vi "Create Weather Display Objects.vi"(8 "Error In":errorcluster, 11 "Display Manager In":refnum<class "Display Manager.lvclass">) -> (0 "Error Out":errorcluster, 3 "Display Manager Out":refnum<class "Display Manager.lvclass">)   [LabVIEW 2021, in "Display Manager.lvclass"]
uses:
  Display Manager.lvclass
  <vilib>/Memosfet/myRIO-Neopixel/RT/Display Utilities/Public/Controls/2D Coordinates.ctl
  <vilib>/Memosfet/myRIO-Neopixel/RT/String/String.lvclass
  C:/Program Files (x86)/National Instruments/LabVIEW 2021/vi.lib/Memosfet/myRIO-Neopixel/RT/Display Element/Display Element.lvclass
  Accessors/Display/Get Display.vi
  <vilib>/Memosfet/myRIO-Neopixel/RT/Display/Display.lvclass
  <vilib>/Memosfet/myRIO-Neopixel/RT/Display Utilities/Display Utilities.lvlib
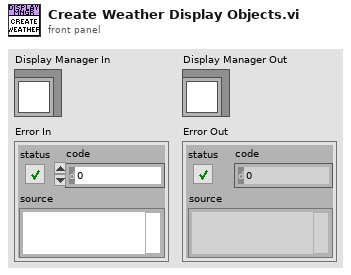
[diagram p1: front panel]
types:
  T1 = typedef "Display Utilities.lvlib/2D Coordinates.ctl" = cluster{"X":i32, "Y":i32}
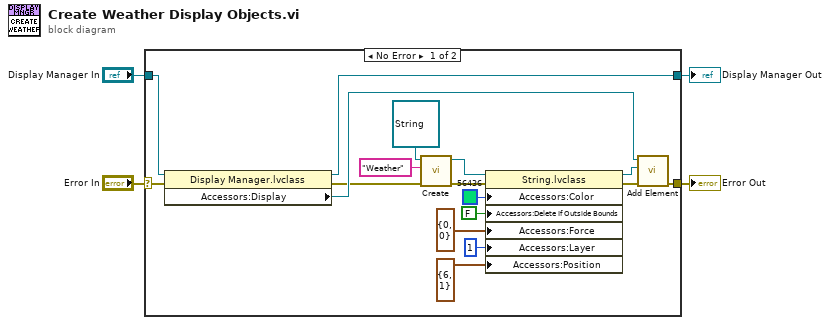
[diagram p0: block diagram]
diagram:
  n1 = case shown="No Error" "Error In" {
    selector: "Error In" -> [w20 w23]
    tunnel: [w6 w23] -> w3
    tunnel: "Display Manager In" -> [w21 w22]
    tunnel: [w17 w22] -> w1
    frame No Error {
      n2 = property class="Display Manager.lvclass"(reference=w21, error in=w20) -> (reference out=w17:refnum<class "Display Manager.lvclass">, error out=w18:errorcluster, "Accessors:Display"=w19:refnum<class "Display.lvclass">)
      n3 = call-dynamic "Create.vi"("Error In"=w18, "Tag"="Weather", "Pixel In"=refnum<class "String.lvclass"> refnum) -> ("Error Out"=w14:errorcluster, "Pixel Out"=w15:refnum<class "String.lvclass">)  [unwired: 7 in]
      n4 = property class="String.lvclass"(reference=w15, error in=w14, "Accessors:Color"=u32 56436 ("Color"), "Accessors:Delete If Outside Bounds"=FALSE ("Delete If Outside Bounds"), "Accessors:Force"=T1 {"X"=0, "Y"=0} ("Force"), "Accessors:Layer"=u32 1 ("Layer"), "Accessors:Position"=T1 {"X"=6, "Y"=1} ("Position")) -> (reference out=w8:refnum<class "String.lvclass">, error out=w7:errorcluster)
      n5 = call <vilib>:"Add Element.vi"("Error In"=w7, "New Element"=w8, "Display In"=w19) -> ("Error Out"=w6:errorcluster)  [unwired: 7 in, 1 out]
    }
    frame Error {
    }
  }
  "Display Manager Out" <- w1
  "Error Out" <- w3
